vi "top player court segment(SubVI).vi"(10 "Top player position":cluster{"Numeric":dbl, "Numeric":dbl}[](array[cluster]), 11 "previous segment":i32) -> (2 "Top player segment position":string)   [LabVIEW 2014]
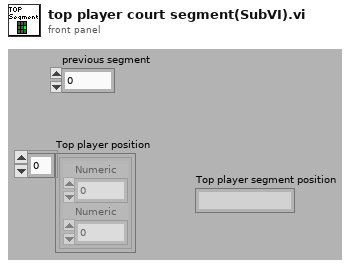
[diagram p1: front panel]
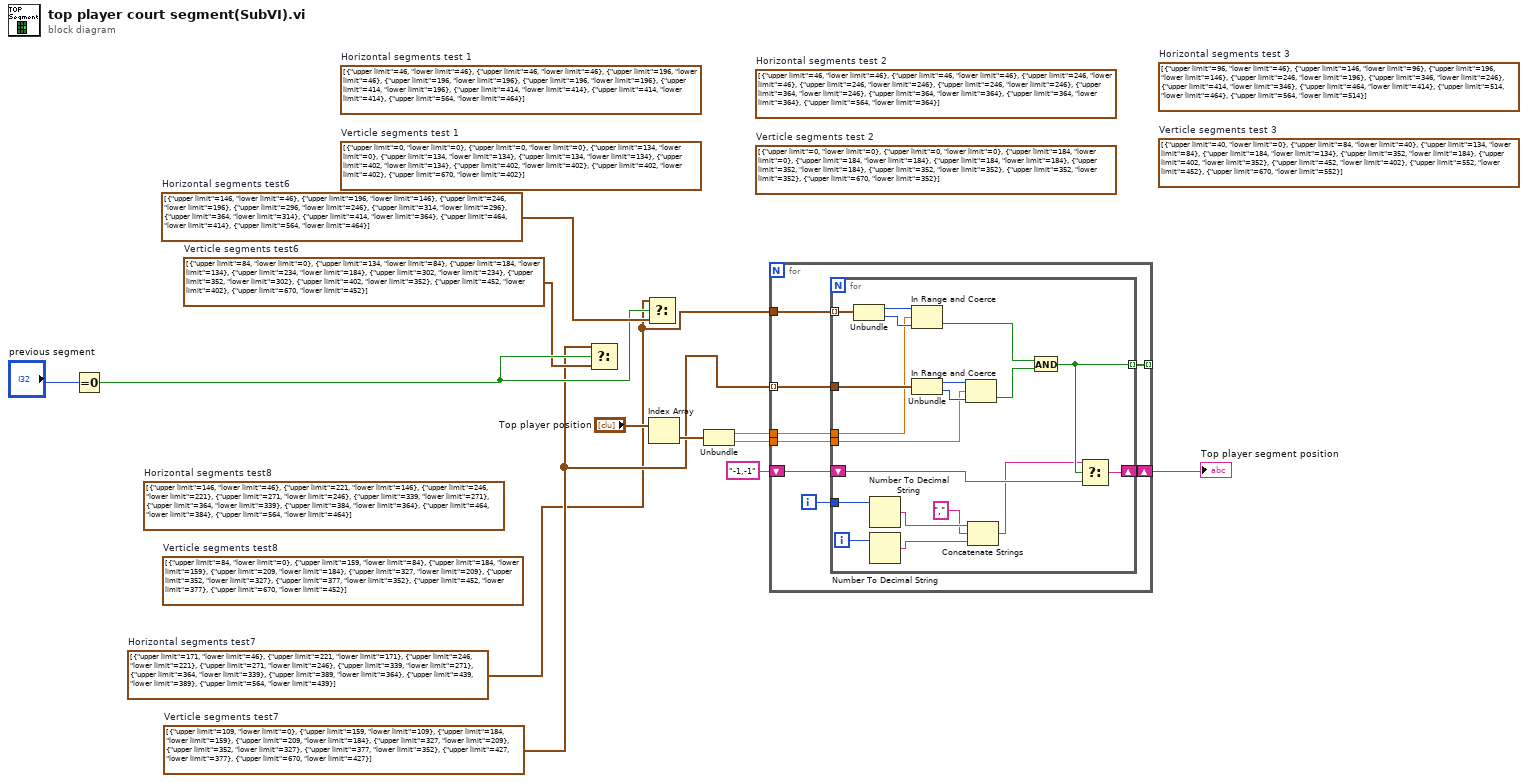
[diagram p0: block diagram]
diagram:
  (unwired) cluster{"upper limit":i32, "lower limit":i32}[] [{"upper limit"=146, "lower limit"=46}, {"upper limit"=221, "lower limit"=146}, {"upper limit"=246, "lower limit"=221}, {"upper limit"=271, "lower limit"=246}, {"upper limit"=339, "lower limit"=271}, {"upper limit"=364, "lower limit"=339}, {"upper limit"=384, "lower limit"=364}, {"upper limit"=464, "lower limit"=384}, {"upper limit"=564, "lower limit"=464}]  # Horizontal segments test8
  (unwired) cluster{"upper limit":i32, "lower limit":i32}[] [{"upper limit"=84, "lower limit"=0}, {"upper limit"=159, "lower limit"=84}, {"upper limit"=184, "lower limit"=159}, {"upper limit"=209, "lower limit"=184}, {"upper limit"=327, "lower limit"=209}, {"upper limit"=352, "lower limit"=327}, {"upper limit"=377, "lower limit"=352}, {"upper limit"=452, "lower limit"=377}, {"upper limit"=670, "lower limit"=452}]  # Verticle segments test8
  w1 = cluster{"upper limit":i32, "lower limit":i32}[] [{"upper limit"=171, "lower limit"=46}, {"upper limit"=221, "lower limit"=171}, {"upper limit"=246, "lower limit"=221}, {"upper limit"=271, "lower limit"=246}, {"upper limit"=339, "lower limit"=271}, {"upper limit"=364, "lower limit"=339}, {"upper limit"=389, "lower limit"=364}, {"upper limit"=439, "lower limit"=389}, {"upper limit"=564, "lower limit"=439}]  # Horizontal segments test7
  w2 = cluster{"upper limit":i32, "lower limit":i32}[] [{"upper limit"=109, "lower limit"=0}, {"upper limit"=159, "lower limit"=109}, {"upper limit"=184, "lower limit"=159}, {"upper limit"=209, "lower limit"=184}, {"upper limit"=327, "lower limit"=209}, {"upper limit"=352, "lower limit"=327}, {"upper limit"=377, "lower limit"=352}, {"upper limit"=427, "lower limit"=377}, {"upper limit"=670, "lower limit"=427}]  # Verticle segments test7
  w5 = cluster{"upper limit":i32, "lower limit":i32}[] [{"upper limit"=146, "lower limit"=46}, {"upper limit"=196, "lower limit"=146}, {"upper limit"=246, "lower limit"=196}, {"upper limit"=296, "lower limit"=246}, {"upper limit"=314, "lower limit"=296}, {"upper limit"=364, "lower limit"=314}, {"upper limit"=414, "lower limit"=364}, {"upper limit"=464, "lower limit"=414}, {"upper limit"=564, "lower limit"=464}]  # Horizontal segments test6
  w3 = cluster{"upper limit":i32, "lower limit":i32}[] [{"upper limit"=84, "lower limit"=0}, {"upper limit"=134, "lower limit"=84}, {"upper limit"=184, "lower limit"=134}, {"upper limit"=234, "lower limit"=184}, {"upper limit"=302, "lower limit"=234}, {"upper limit"=352, "lower limit"=302}, {"upper limit"=402, "lower limit"=352}, {"upper limit"=452, "lower limit"=402}, {"upper limit"=670, "lower limit"=452}]  # Verticle segments test6
  (unwired) cluster{"upper limit":i32, "lower limit":i32}[] [{"upper limit"=0, "lower limit"=0}, {"upper limit"=0, "lower limit"=0}, {"upper limit"=184, "lower limit"=0}, {"upper limit"=184, "lower limit"=184}, {"upper limit"=184, "lower limit"=184}, {"upper limit"=352, "lower limit"=184}, {"upper limit"=352, "lower limit"=352}, {"upper limit"=352, "lower limit"=352}, {"upper limit"=670, "lower limit"=352}]  # Verticle segments test 2
  (unwired) cluster{"upper limit":i32, "lower limit":i32}[] [{"upper limit"=46, "lower limit"=46}, {"upper limit"=46, "lower limit"=46}, {"upper limit"=246, "lower limit"=46}, {"upper limit"=246, "lower limit"=246}, {"upper limit"=246, "lower limit"=246}, {"upper limit"=364, "lower limit"=246}, {"upper limit"=364, "lower limit"=364}, {"upper limit"=364, "lower limit"=364}, {"upper limit"=564, "lower limit"=364}]  # Horizontal segments test 2
  (unwired) cluster{"upper limit":i32, "lower limit":i32}[] [{"upper limit"=0, "lower limit"=0}, {"upper limit"=0, "lower limit"=0}, {"upper limit"=134, "lower limit"=0}, {"upper limit"=134, "lower limit"=134}, {"upper limit"=134, "lower limit"=134}, {"upper limit"=402, "lower limit"=134}, {"upper limit"=402, "lower limit"=402}, {"upper limit"=402, "lower limit"=402}, {"upper limit"=670, "lower limit"=402}]  # Verticle segments test 1
  (unwired) cluster{"upper limit":i32, "lower limit":i32}[] [{"upper limit"=46, "lower limit"=46}, {"upper limit"=46, "lower limit"=46}, {"upper limit"=196, "lower limit"=46}, {"upper limit"=196, "lower limit"=196}, {"upper limit"=196, "lower limit"=196}, {"upper limit"=414, "lower limit"=196}, {"upper limit"=414, "lower limit"=414}, {"upper limit"=414, "lower limit"=414}, {"upper limit"=564, "lower limit"=464}]  # Horizontal segments test 1
  (unwired) cluster{"upper limit":i32, "lower limit":i32}[] [{"upper limit"=40, "lower limit"=0}, {"upper limit"=84, "lower limit"=40}, {"upper limit"=134, "lower limit"=84}, {"upper limit"=184, "lower limit"=134}, {"upper limit"=352, "lower limit"=184}, {"upper limit"=402, "lower limit"=352}, {"upper limit"=452, "lower limit"=402}, {"upper limit"=552, "lower limit"=452}, {"upper limit"=670, "lower limit"=552}]  # Verticle segments test 3
  (unwired) cluster{"upper limit":i32, "lower limit":i32}[] [{"upper limit"=96, "lower limit"=46}, {"upper limit"=146, "lower limit"=96}, {"upper limit"=196, "lower limit"=146}, {"upper limit"=246, "lower limit"=196}, {"upper limit"=346, "lower limit"=246}, {"upper limit"=414, "lower limit"=346}, {"upper limit"=464, "lower limit"=414}, {"upper limit"=514, "lower limit"=464}, {"upper limit"=564, "lower limit"=514}]  # Horizontal segments test 3
  n1 = Equal To 0?(x="previous segment") -> (x = 0?=w4:bool)
  n2 = Select(t=w2, s=w4, f=w3) -> ()  [unwired: 1 out]
  n3 = Select(t=w1, s=w4, f=w5) -> ()  [unwired: 1 out]
  n4 = Index Array(array="Top player position") -> (element=w11:cluster{"Numeric":dbl, "Numeric":dbl})  [unwired: 1 in]
  n5 = Unbundle(w11) -> ("Numeric"=w9:dbl, "Numeric"=w10:dbl)
  n6 = for {
    tunnel: w2 -> [w19] mode=indexing
    tunnel: w1 -> [w20]
    tunnel: w10 -> [w18]
    tunnel: w9 -> [w17]
    tunnel: [w16] -> _ mode=indexing
    shift-right: [w14] -> w7
    shift-left: "-1,-1" ("decimal integer string") -> [w13]
    i -> [w15]
    n7 = for {
      tunnel: w20 -> [w39] mode=indexing
      tunnel: w19 -> [w38]
      tunnel: w18 -> [w33]
      tunnel: w17 -> [w32]
      tunnel: [w29] -> w16 mode=indexing
      tunnel: w15 -> [w26]
      shift-right: [w28] -> w14
      shift-left: w13 -> [w27]
      i -> [w25]
      n8 = Unbundle(w39) -> ("upper limit"=w37:i32, "lower limit"=w36:i32)
      n9 = Number To Decimal String(number=w26) -> (decimal integer string=w24:string)  [unwired: 1 in]
      n10 = Number To Decimal String(number=w25) -> (decimal integer string=w22:string)  [unwired: 1 in]
      n11 = In Range and Coerce(upper limit=w37, x=w32, lower limit=w36) -> (In Range?=w31:bool)  [unwired: 1 out]
      n12 = Unbundle(w38) -> ("upper limit"=w35:i32, "lower limit"=w34:i32)
      n13 = In Range and Coerce(upper limit=w35, x=w33, lower limit=w34) -> (In Range?=w30:bool)  [unwired: 1 out]
      n14 = Concatenate Strings(w24, "," ("string"), w22) -> (w23:string)
      n15 = And(x=w31, y=w30) -> (x .and. y?=w29:bool)
      n16 = Select(t=w23, s=w29, f=w27) -> (s? t:f=w28:string)
    }
  }
  "Top player segment position" <- w7
